vi "ProcessHealthAndStatusUpdates.vi"(11 "HealthAndStatusSettings":T1={"InternalHealthAndStatusFIFO"="InternalHealthAndStatusFIFO", "HealthAndStatusQueryFIFO"="HealthAndStatusQueryFIFO", "HealthAndStatusResponseFIFO"="HealthAndStatusResponseFIFO", "HealthAndStatusMemory"="HealthAndStatusMemory", "MemorySize"=0}) -> ()   [LabVIEW 2016, in "FPGAHealthAndStatus.lvlib"]
uses:
  FPGAHealthAndStatus.lvlib
  DataTypes/HealthAndStatusSettings.ctl
  <vilib>/rvi/Emulation/niFpgaGetClockAttributes.vi
  <vilib>/rvi/Emulation/niFpgaSctlEmulationGetInTimedLoop.vi
  <vilib>/rvi/Emulation/niFpgaEmulationReportErrorSimple.vi
  <vilib>/rvi/DataTransferAndStorage/Container/Common/niFpgaContainerExecOnDevCompGetState.vi
  <vilib>/rvi/Emulation/niFpgaEmulationIsFPGAContextNoSignature.vi
  <vilib>/rvi/errors/niFpgaSetErrorForExecOnDevCompSimple.vi
  <vilib>/rvi/eio/common/nirviEmuReportErrorAndStop.vi
  <vilib>/rvi/DataTransferAndStorage/Container/Common/niFpgaContainerGetUniqueNameForEmu.vi
  <vilib>/rvi/FIFO/Fifo_Resource/nirvififoEmulationSetSize.vi
  <vilib>/rvi/FIFO/Fifo_Resource/nirviFifoEmulationQueueMgr.vi
  <instcachedir>/0/nirviFifoEmulationQueueMgr_E5CAEC123FF24DC58D834DCA3CDAA9B5.lvgen/nirviFifoEmulationQueueMgr_E5CAEC123FF24DC58D834DCA3CDAA9B5_011.vi
  <vilib>/rvi/FIFO/Fifo_Resource/nirvififoEmulationDetermineInputValidOut.vi
  <vilib>/rvi/FIFO/Fifo_Resource/nirvififoEmulationCreateLock.vi
  <vilib>/rvi/Emulation/niFpgaProcessEmulError.vi
  <vilib>/rvi/FIFO/Fifo_Resource/nirvififoEmulationObtainLock.vi
  <vilib>/rvi/FIFO/Fifo_Resource/nirvififoEmulationReleaseLock.vi
  <vilib>/rvi/occurrence/nirviWaitOnOccurrenceBase.vi
  <vilib>/rvi/errors/nirviReportUnexpectedCaseInternalError.vi
  <vilib>/rvi/errors/nirviReportUnexpectedCaseInternalError (U32).vi
  <vilib>/Utility/error.llb/Clear Errors.vi
  <vilib>/rvi/interface/RandomDataEmulation/niFpgaRandomDataHandleErrors.vi
  <vilib>/rvi/Memory/Memory_Emulation/niFpgaMemoryEmulationCacheClearOnFirstRun.vi
  <vilib>/rvi/Memory/Memory_Emulation/nirvimemoryEmulationManagerCache_MakeExclusive.vi
  <vilib>/rvi/Memory/Memory_Emulation/niFpgaMemoryEmulationValidateCache.vi
  <vilib>/rvi/Memory/Memory_Emulation/nirvimemoryEmulationManagerCache_InsertValue.vi
  <vilib>/rvi/Memory/Memory_Emulation/nirvimemoryEmulationManagerCache_ReleaseExclusive.vi
  <vilib>/rvi/Memory/Memory_Emulation/nirvimemoryEmulationManagerCache_GetValue.vi
  <vilib>/rvi/Memory/Memory_Emulation/nirvimemoryEmulationManagerCache_SetValue.vi
  <vilib>/rvi/Emulation/niFpgaSctlEmulationResourceMgr.vi
  <vilib>/rvi/Emulation/niFpgaCriticalErrorInLSC.vi
  <vilib>/rvi/DataTransferAndStorage/Container/XNode/niFpgaContainer.xnode
  <vilib>/rvi/FIFO/Fifo_Resource/niFpgaFifoEmulationRefIn.vi
  <vilib>/rvi/Memory/Memory_Emulation/niFpgaMemoryEmulationRefIn.vi
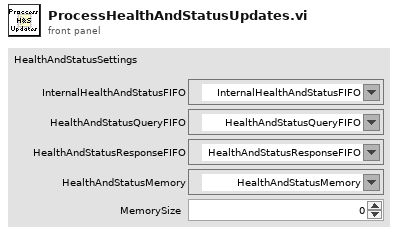
[diagram p1: front panel]
types:
  T1 = typedef "FPGAHealthAndStatus.lvlib/HealthAndStatusSettings.ctl" = cluster{"InternalHealthAndStatusFIFO":refnum<k21>, "HealthAndStatusQueryFIFO":refnum<k21>, "HealthAndStatusResponseFIFO":refnum<k21>, "HealthAndStatusMemory":refnum<k21>, "MemorySize":i32}
  T2 = cluster{"Address":u32, "UpdateMode":enum8{"NOP", "Set", "Add", "Subtract", "Or"}, "Data":u64}
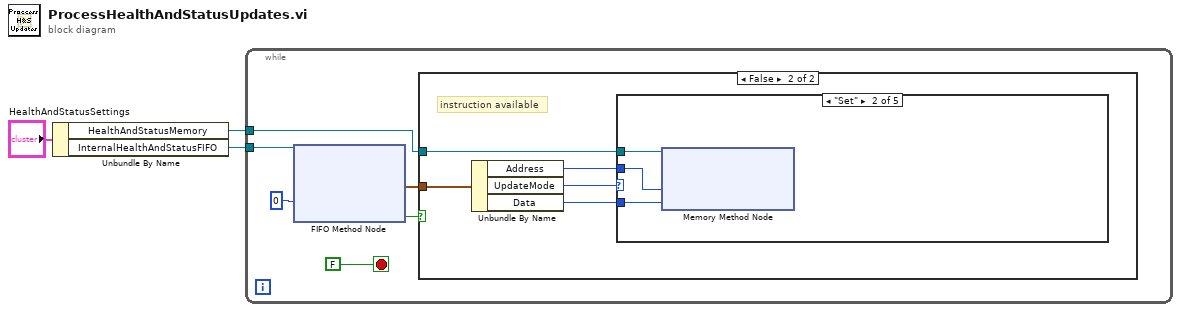
[diagram p0: block diagram]
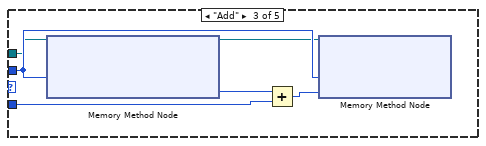
[diagram p4: hidden frame]
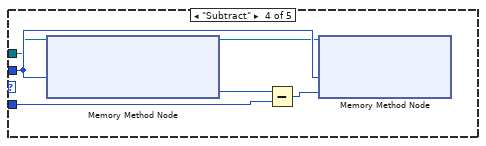
[diagram p5: hidden frame]
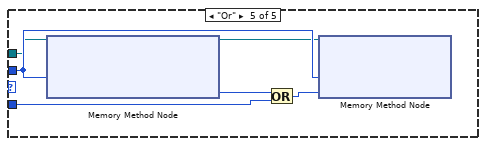
[diagram p6: hidden frame]
diagram:
  n1 = Unbundle By Name("HealthAndStatusSettings") -> ("HealthAndStatusMemory"=w1:refnum<k21>, "InternalHealthAndStatusFIFO"=w2:refnum<k21>)
  n2 = while {
    tunnel: w2 -> [w5]
    tunnel: w1 -> [w4]
    stop <- FALSE stop-if-true
    n3 = xnode ("FIFO Method Node")("Timeout"=0, "FIFO In"=w5) -> ("Element"=w7:T2, "Timed Out?"=w8:bool)  [unwired: 1 out]
    n4 = case shown="False" w8 {
      tunnel: w7 -> [_ w14]
      tunnel: w4 -> [_ w10]
      frame True {
        # "no instruction available"
      }
      frame False {
        # "instruction available"
        n5 = Unbundle By Name(w14) -> ("Address"=w12:u32, "UpdateMode"=w13:enum8{"NOP", "Set", "Add", "Subtract", "Or"}, "Data"=w11:u64)
        n6 = case shown="\"Set\"" w13 {
          tunnel: w12 -> [_ w17 w22 w28 w34]
          tunnel: w11 -> [_ w16 w20 w26 w32]
          tunnel: w10 -> [_ w15 w19 w25 w31]
          frame "NOP", Default {
          }
          frame "Set" {
            n7 = xnode ("Memory Method Node")("Address"=w17, "Data"=w16, "Memory In"=w15) -> ()  [unwired: 1 out]
          }
          frame "Add" {
            n8 = xnode ("Memory Method Node")("Address"=w22, "Memory In"=w19) -> ("Data"=w23:u64, "Memory Out"=w18:refnum<k21>)
            n9 = Add(x=w23, y=w20) -> (x+y=w21:u64)
            n10 = xnode ("Memory Method Node")("Address"=w22, "Data"=w21, "Memory In"=w18) -> ()  [unwired: 1 out]
          }
          frame "Subtract" {
            n11 = xnode ("Memory Method Node")("Address"=w28, "Memory In"=w25) -> ("Data"=w29:u64, "Memory Out"=w24:refnum<k21>)
            n12 = Subtract(x=w29, y=w26) -> (x-y=w27:u64)
            n13 = xnode ("Memory Method Node")("Address"=w28, "Data"=w27, "Memory In"=w24) -> ()  [unwired: 1 out]
          }
          frame "Or" {
            n14 = xnode ("Memory Method Node")("Address"=w34, "Memory In"=w31) -> ("Data"=w35:u64, "Memory Out"=w30:refnum<k21>)
            n15 = Or(x=w35, y=w32) -> (x .or. y?=w33:u64)
            n16 = xnode ("Memory Method Node")("Address"=w34, "Data"=w33, "Memory In"=w30) -> ()  [unwired: 1 out]
          }
        }
      }
    }
  }
